vi "AddPolarVectors.vi"(9 "Angle2":dbl[](array[numeric]), 10 "Angle1":dbl[](array[numeric]), 11 "Magnitude":dbl[](array[numeric])) -> (1 "New Angle2":dbl, 2 "New Angle1":dbl, 3 "New Magnitude":dbl)   [LabVIEW 2014]
uses:
  <vilib>/Analysis/coordinate.llb/3D Coordinate Conversion (Array).vi
  <vilib>/Analysis/coordinate.llb/3D Coordinate Conversion (Scalar).vi
  <vilib>/Analysis/NI_AALPro.lvlib
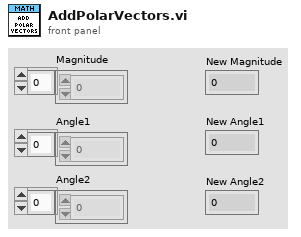
[diagram p1: front panel]
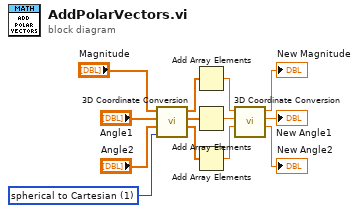
[diagram p0: block diagram]
diagram:
  w13 = u16 1 items=["Cartesian to spherical", "spherical to Cartesian", "Cartesian to cylindrical", "cylindrical to Cartesian", "spherical to cylindrical", "cylindrical to spherical"] ("conversion type")
  n1 = call-poly <vilib>:"3D Coordinate Conversion.vi"("conversion type"=w13, "Axis 3"="Angle2", "Axis 2"="Angle1", "Axis 1"="Magnitude") -> ("Axis 3 Out"=w9:dbl[], "Axis 2 Out"=w8:dbl[], "Axis 1 Out"=w7:dbl[])  [unwired: 4 in, 1 out]
  n2 = Add Array Elements(numeric array=w7) -> (sum=w4:dbl)
  n3 = Add Array Elements(numeric array=w8) -> (sum=w5:dbl)
  n4 = Add Array Elements(numeric array=w9) -> (sum=w6:dbl)
  n5 = call-poly <vilib>:"3D Coordinate Conversion.vi"("axis 3"=w6, "axis 2"=w5, "axis 1"=w4) -> ("axis 3 out"=→"New Angle2":dbl, "axis 2 out"=→"New Angle1":dbl, "axis 1 out"=→"New Magnitude":dbl)  [unwired: 5 in, 1 out]
